vi "get_timestamp.vi"(8 "error in (no error)":errorcluster, 11 "Index":i32) -> (0 "error out":errorcluster, 3 "Signal Array":T1[](array[typedef]))   [LabVIEW 2012]
uses:
  Public API/Post_Signal.ctl
  Role ID.ctl
  Hardware ID.ctl
  <vilib>/addons/database/Auxilliary.llb/DB Tools Cursor Type.ctl
  <vilib>/addons/database/Connection.llb/Conn Execute.vi
  <vilib>/addons/database/Recordset.llb/Rec Fetch Recordset Data (R).vi
  <vilib>/addons/database/Recordset.llb/Rec Destroy - Connection.vi
  <vilib>/addons/database/_DB Variant To Data/Database Variant To Data.xnode
  <vilib>/addons/database/NI_Database_API.lvlib
panel:
  out "SQL Query Sintax":string
  # "Signal"
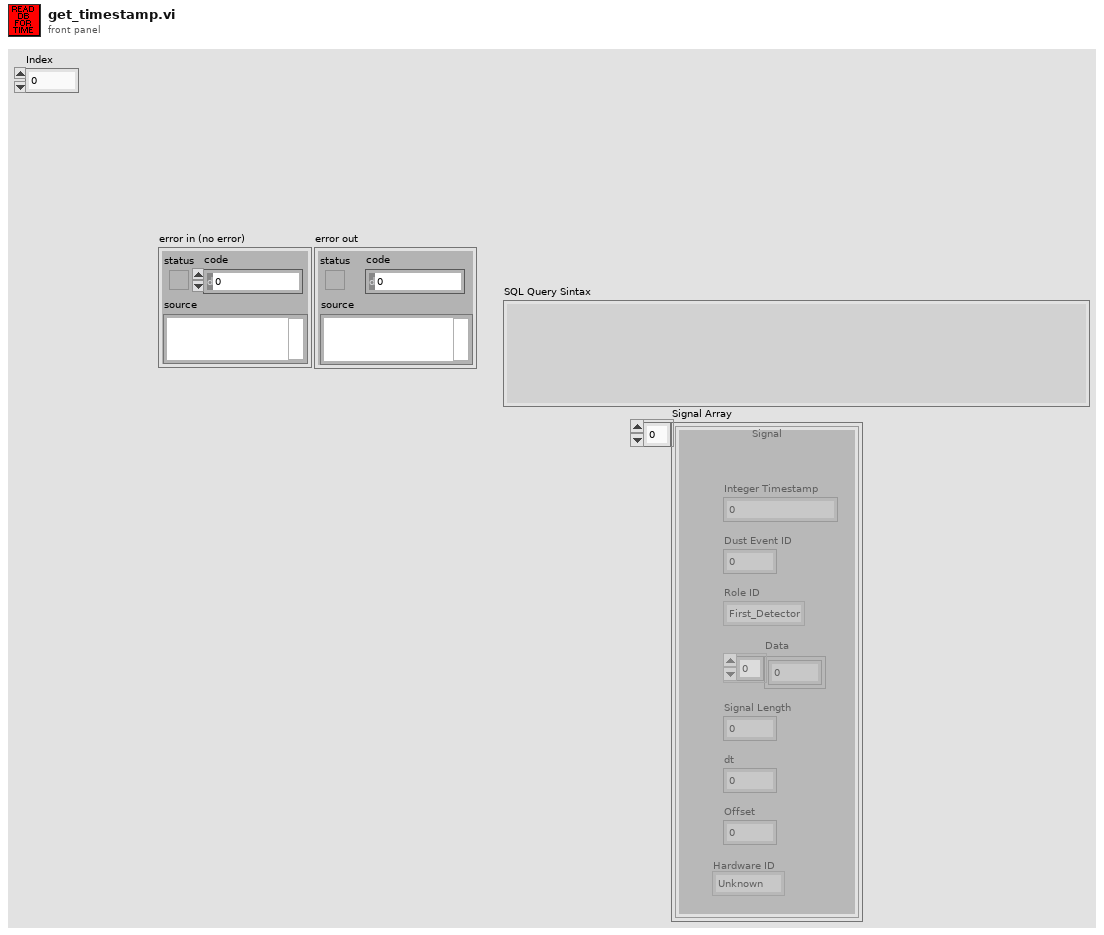
[diagram p1: front panel]
types:
  T1 = typedef "Post_Signal.ctl" = cluster{"Integer Timestamp":i64, "Dust Event ID":i64, "Role ID":T2, "Data":sgl[], "Signal Length":i32, "dt":sgl, "Offset":dbl, "Hardware ID":T3}
  T2 = typedef "Role ID.ctl" = enum16{"First_Detector", "Second_Detector", "Third_Detector", "LeCroy_CH1", "LeCroy_CH2", "LeCroy_CH3", "LeCroy_CH4", "PSU"}
  T3 = typedef "Hardware ID.ctl" = enum16{"Unknown", "CSA 1", "CSA 2", "CSA 3", "CSA 4", "CSA 5", "CSA 6"}
  T4 = typedef "NI_Database_API.lvlib/DB Tools Cursor Type.ctl" = enum16{"forward-only", "keyset", "dynamic", "static"}
  T5 = typedef "NI_Database_API.lvlib/Conn ObjectReference.ctl" = refnum<k1>
  T6 = typedef "NI_Database_API.lvlib/Rec ObjectReference.ctl" = refnum<k1>
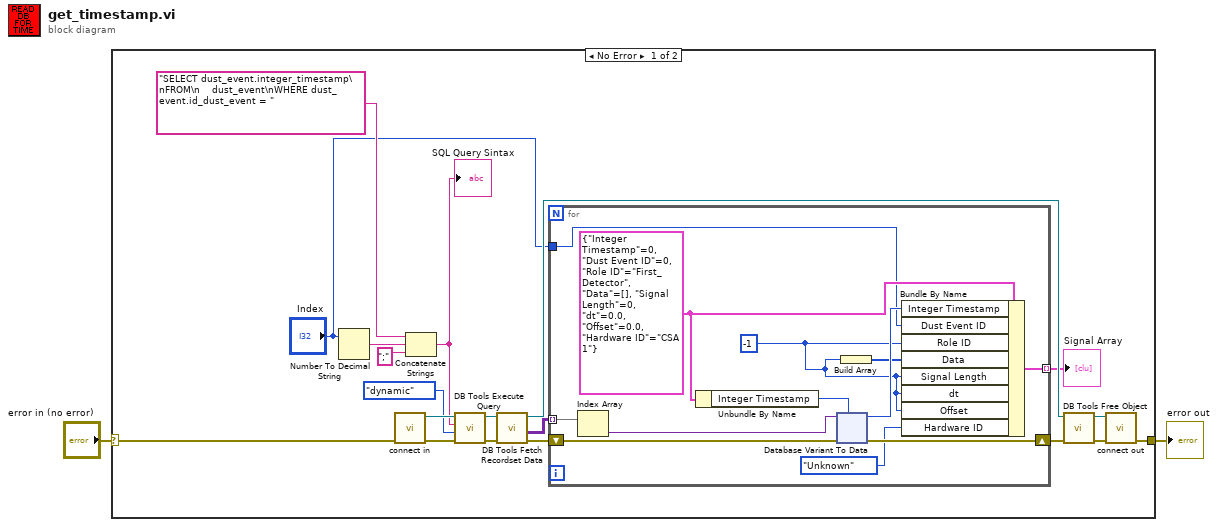
[diagram p0: block diagram]
diagram:
  n1 = case shown="No Error" "error in (no error)" {
    selector: "error in (no error)" -> [w9 w66]
    tunnel: [w11 w66] -> w1
    frame No Error {
      n2 = Number To Decimal String(number="Index") -> (decimal integer string=w8:string)  [unwired: 1 in]
      n3 = call "connect in.vi"("error in (no error)"=w9) -> ("error out"=w17:errorcluster, "Database Connection"=w18:T5)  [unwired: 6 in, 1 out]
      n4 = Concatenate Strings("SELECT dust_event.integer_timestamp\nFROM\n    dust_event\nWHERE dust_event.id_dust_event = " ("string"), w8, ";" ("string")) -> (w12:string)
      "SQL Query Sintax" <- w12
      n5 = call-poly <vilib>:"DB Tools Execute Query.vi"("error in (no error)"=w17, "cursor type"=DB_Tools_Cursor_Type."dynamic", "SQL query"=w12, "connection reference"=w18) -> ("error out"=w20:errorcluster, "recordset reference"=w21:T6)  [unwired: 4 in]
      n6 = call-poly <vilib>:"DB Tools Fetch Recordset Data.vi"("error in (no error)"=w20, "recordset reference"=w21) -> ("error out"=w7:errorcluster, "recordset data"=w5:variant[][], "recordset reference out"=w19:T6)  [unwired: 3 in]
      n7 = for {
        tunnel: w5 -> [w27] mode=indexing
        shift-right: [w32] -> w6
        shift-left: w7 -> [w33]
        tunnel: [w26] -> w4 mode=indexing
        tunnel: "Index" -> [w24]
        w22 = i64 -1 ("Dust Event ID")
        w30 = T1 {"Integer Timestamp"=0, "Dust Event ID"=0, "Role ID"=enum."First_Detector", "Data"=[], "Signal Length"=0, "dt"=0.0, "Offset"=0.0, "Hardware ID"=enum."CSA 1"} ("Post_Signal")
        n8 = Index Array(array=w27) -> (element=w28:variant)  [unwired: 1 in]
        n9 = Unbundle By Name(w30) -> ("Integer Timestamp"=w29:i64)
        n10 = xnode "Database Variant To Data"("database variant"=w28, "error in"=w33, "type"=w29) -> ("data"=w31:i64, "error out"=w32:errorcluster)
        n11 = Build Array(w22) -> (w23:i64[])
        n12 = Bundle By Name(cluster=w30, "Integer Timestamp"=w31, "Dust Event ID"=w24, "Role ID"=w22, "Data"=w23, "Signal Length"=w22, "dt"=w22, "Offset"=w22, "Hardware ID"=Hardware_ID."Unknown") -> (w26:T1)
      }
      "Signal Array" <- w4
      n13 = call-poly <vilib>:"DB Tools Free Object.vi"("error in (no error)"=w6, "recordset reference"=w19) -> ("error out"=w14:errorcluster, "connection reference"=w16:T5)  [unwired: 8 in]
      n14 = call "connect out.vi"("error in (no error)"=w14, "connection reference"=w16) -> ("error out"=w11:errorcluster)  [unwired: 9 in]
    }
    frame Error {
    }
  }
  "error out" <- w1
